vi "SetDefaultCellStyles.vi"(8 "error in (no error)":errorcluster, 9 "Defautl Style":T1(ring), 10 "CellStyle.lvclass":refnum<class "CellStyle.lvclass">, 11 "DataGridView in":refnum<class "DataGridView.lvclass">) -> (0 "error out":errorcluster, 3 "DataGridView out":refnum<class "DataGridView.lvclass">)   [LabVIEW 2013, in "DataGrid.lvlib" / "DataGridView.lvclass"]
doc: "Applies a cell style to any cell, by row and column. If the row is set to -1, it will apply to the column headers.\n\nUse this sparingly, as it can have a very negative effect on performance. Instead, use the DefaultCellStyle and AlternatingRowsDefaultCellStyle"
uses:
  DataGridView.lvclass
  System.Windows.Forms
  CellStyle/CellStyle.lvclass
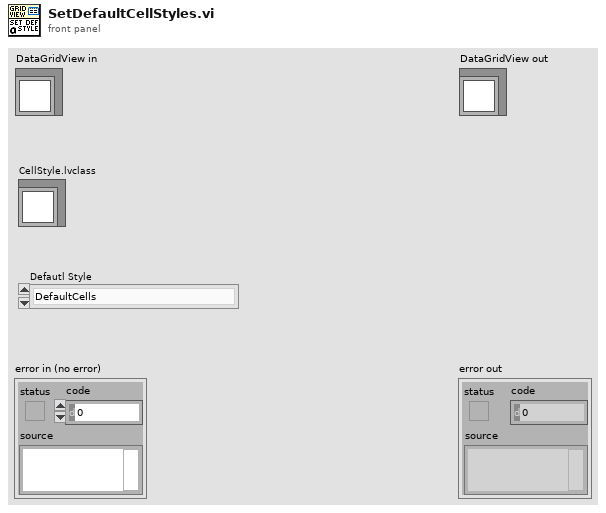
[diagram p1: front panel]
types:
  T1 = enum16{"DefaultCells", "AlternatingRowsDefaultStyle"}
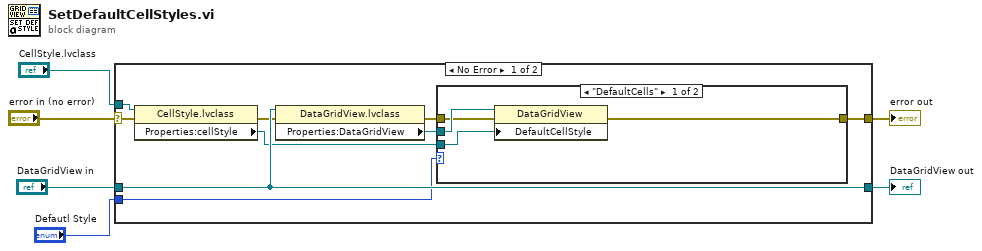
[diagram p0: block diagram]
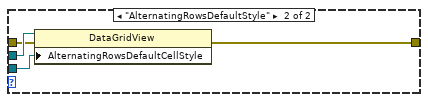
[diagram p2: hidden frame]
diagram:
  n1 = case shown="No Error" "error in (no error)" {
    selector: "error in (no error)" -> [w14 w25]
    tunnel: [w11 w25] -> w5
    tunnel: [w13 w24] -> w3
    tunnel: "DataGridView in" -> [w13 w24]
    tunnel: "CellStyle.lvclass" -> [w15 _]
    tunnel: "Defautl Style" -> [w7 _]
    frame No Error {
      n2 = property class="CellStyle.lvclass"(reference=w15, error in=w14) -> (error out=w12:errorcluster, "Properties:cellStyle"=w8:refnum<k24>)  [unwired: 1 out]
      n3 = property class="DataGridView.lvclass"(reference=w13, error in=w12) -> (error out=w9:errorcluster, "Properties:DataGridView"=w10:refnum<k24>)  [unwired: 1 out]
      n4 = case shown="\"DefaultCells\"" w7 {
        tunnel: [w17 w21] -> w11
        tunnel: w10 -> [w19 w23]
        tunnel: w9 -> [w18 w22]
        tunnel: w8 -> [w16 w20]
        frame "DefaultCells" {
          n5 = property class="DataGridView"(reference=w19, error in=w18, "DefaultCellStyle"=w16) -> (error out=w17:errorcluster)  [unwired: 1 out]
        }
        frame "AlternatingRowsDefaultStyle" {
          n6 = property class="DataGridView"(reference=w23, error in=w22, "AlternatingRowsDefaultCellStyle"=w20) -> (error out=w21:errorcluster)  [unwired: 1 out]
        }
      }
    }
    frame Error {
    }
  }
  "error out" <- w5
  "DataGridView out" <- w3
